vi "tripod gait (forNM)_0916.vi"(0 "data of 5th order formula\nts,tair,a1-a6":dbl[](array[numeric]), 1 "first or second":bool, 3 "buffer ratio":dbl, 4 "t_shift":dbl=0.000125, 5 "sample time":dbl=0.002, 9 "T_ratio":dbl, 10 "initial":bool) -> (7 "R1、R2 at 180":cluster{"1 at 180":bool, "2 at 180":bool}, 8 "reset step(indicator)":bool, 11 "start to calculate power":bool, 12 "output data":bool, 13 "Confirm(indicator)":bool, 14 "now gait info":T1, 15 "t1 out":dbl, 16 "finished":bool, 17 "t2 out":dbl, 18 "SET POINT V":dbl(graph), 19 "start to calculate the cost":bool, 20 "state":dbl, 21 "state 2":dbl, 23 "Set Point":dbl, 24 "Set Point 2":dbl, 25 "step count NM":dbl, 26 "period":dbl, 27 "new data of 5th NM":dbl[](array[numeric]))   [LabVIEW 2019]
panel:
  out "set point 2":dbl(graph)
  out "set point":dbl(graph)
  out "Numeric":dbl
  out "beta":dbl
  # "Nelder Mead"
  # "Input"
  # "Output"
  # "Others"
  # "loop period(ms)"
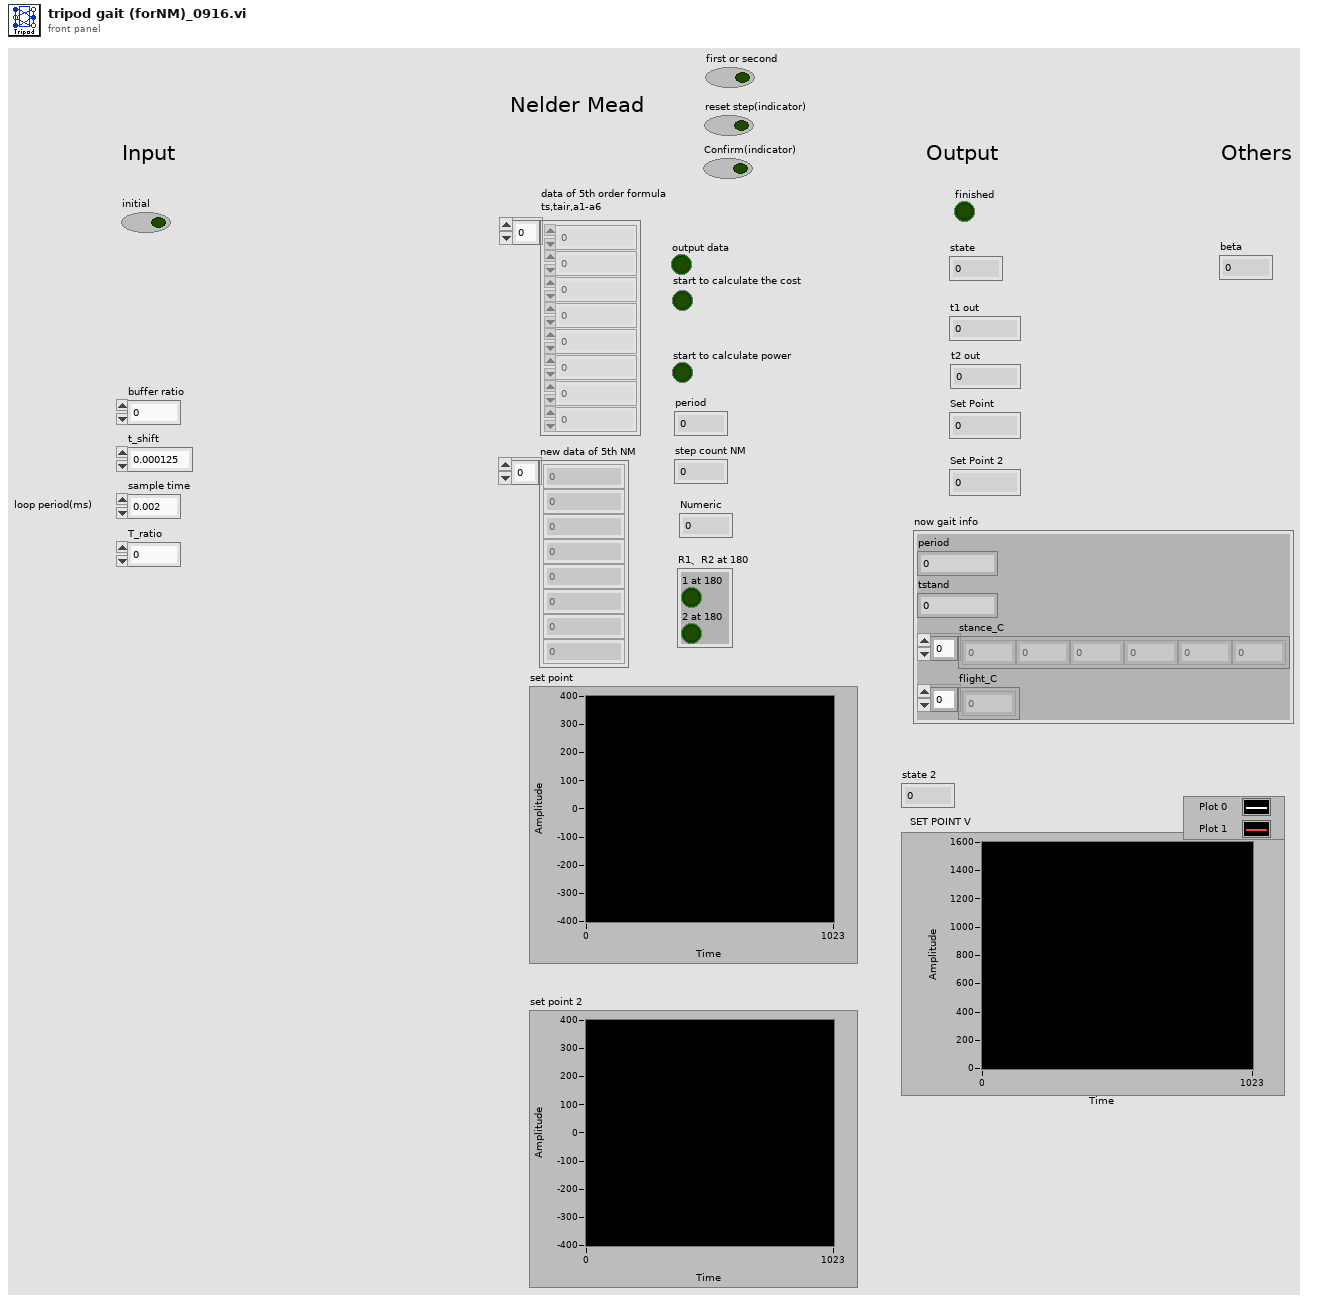
[diagram p1: front panel]
types:
  T1 = cluster{"period":dbl, "tstand":dbl, "stance_C":dbl[], "flight_C":dbl[]}
  T2 = cluster{"output cluster 2":cluster{"period":dbl, "tstand":dbl, "stance_C":dbl[], "flight_C":dbl[]}, "time180":dbl}
  T3 = cluster{"output cluster 2":cluster{"period":dbl, "tstand":dbl, "stance_C":dbl[], "flight_C":dbl[]}, "t2_out":dbl}
  T4 = cluster{"output cluster 2":cluster{"period":dbl, "tstand":dbl, "stance_C":dbl[], "flight_C":dbl[]}, "t1_out":dbl}
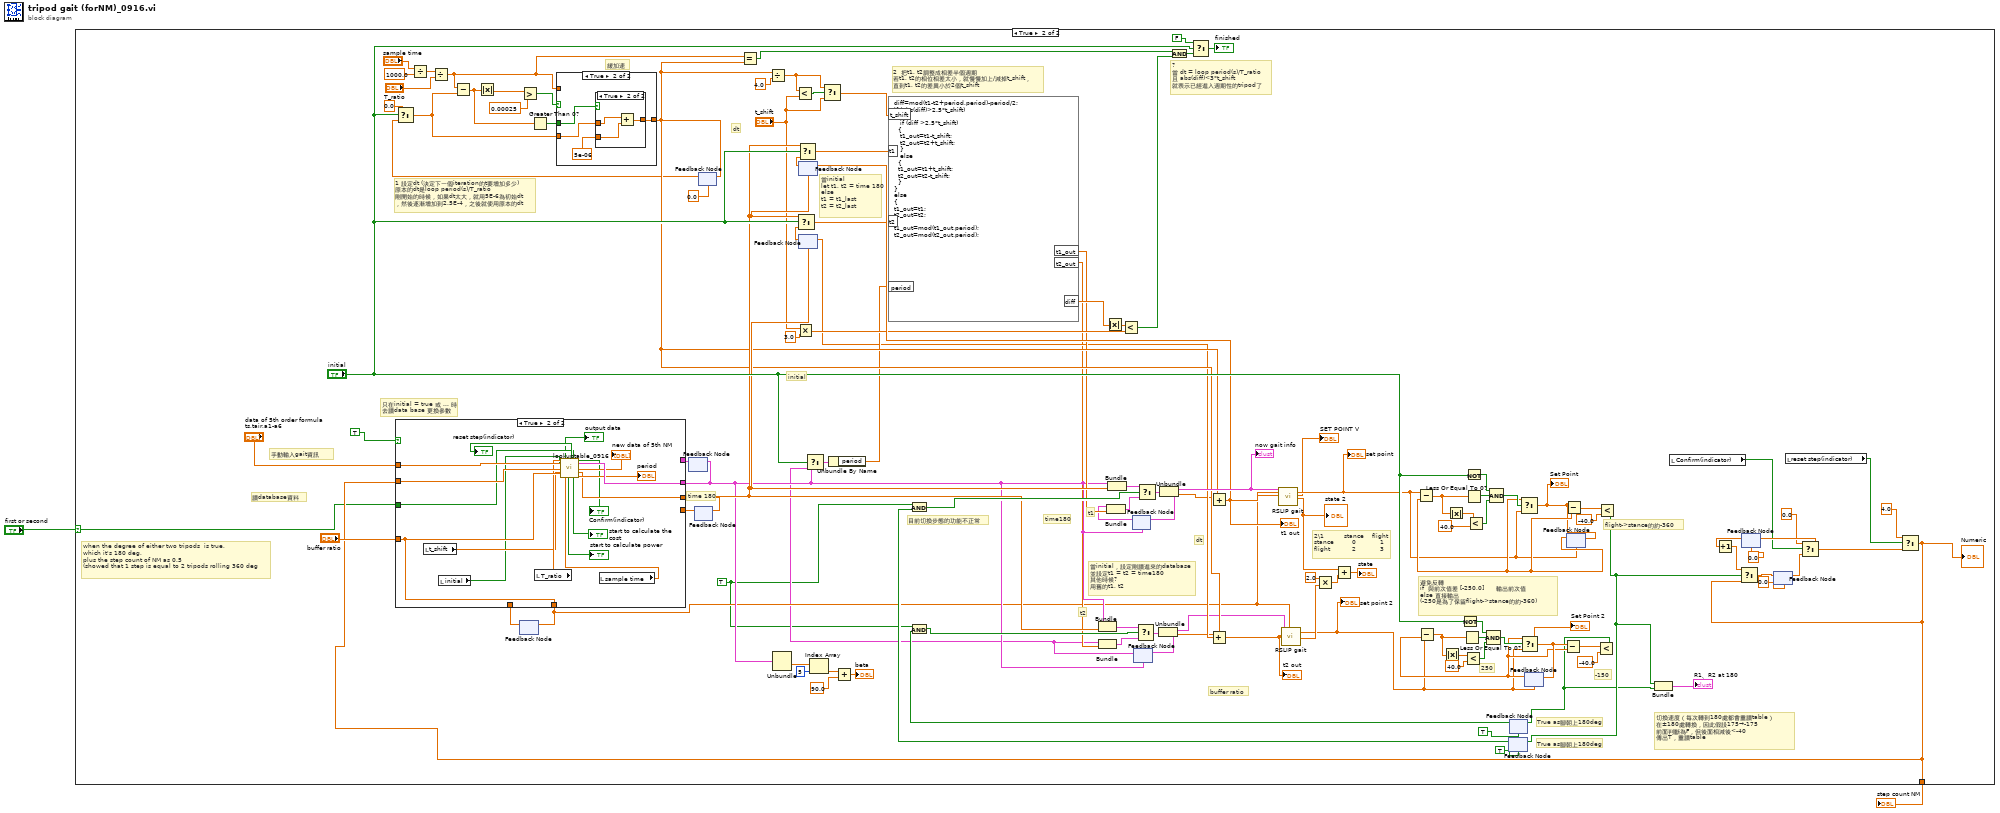
[diagram p0: block diagram]
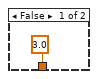
[diagram p2: hidden frame]
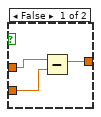
[diagram p4: hidden frame]
diagram:
  n1 = case shown="True" "first or second" {
    selector: "first or second" -> [_ w11]
    tunnel: [3.0 ("t") w13] -> w2
    frame False {
    }
    frame True {
      w31 = TRUE
      # "when the degree of either two tripods  is true, \nwhich it's 180 deg, \nplus the step count of NM as 0.5\n(showed that 1 step is equal to 2 tripods rolling 360 deg"
      # "目前切換步態的功能不正常"
      # "True as腳朝上180deg"
      # "True as腳朝上180deg"
      # "time180"
      # "t2"
      # "t1"
      # "dt"
      # "當initial，設定剛讀進來的database\n並設定t1 = t2 = time180\n其他時候?\n用舊的t1, t2"
      # "當initial\nlet t1, t2 = time 180\nelse\nt1 = t1_last\nt2 = t2_last"
      # "2  把t1, t2調整成相差半個週期\n若t1, t2的相位相差太小，就慢慢加上/減掉t_shift，\n直到t1, t2的差異小於2個t_shift"
      # "只在initial = true 或 ... 時\n去讀data base 更換參數"
      # "?\n當 dt = loop period(s)/T_ratio\n且 abs(diff)<3*t_shift\n就表示已經進入週期性的tripod了"
      # "1 設定dt (決定下一個iteration的t要增加多少)\n原本的dt是loop period(s)/T_ratio\n剛開始的時候，如果dt太大，就用5E-6為初始dt\n，然後逐漸增加到2.5E-4，之後就使用原本的dt"
      # "dt"
      # "initial"
      # "time 180"
      # "緩加速"
      # "切換速度（每次轉到180處都會重讀table）\n在±180處轉換，因此假設175→-175\n前面判斷為F，但後面相減後<-40\n傳出T，重讀table"
      # "手動輸入gait資訊"
      # "-150"
      # "250"
      # "buffer ratio"
      # "讀database資料"
      # "flight->stance的約-360"
      # "避免反轉\nif  與前次值差 [-250,0]      輸出前次值 \nelse 直接輸出\n(-250是為了保留flight->stance的約-360)"
      # "2\\1          stance    flight\nstance         0            1\nflight           2            3"
      n2 = Divide(x="sample time", y=1000.0) -> (x/y=w85:dbl)
      n3 = Divide(x=w85, y="T_ratio") -> (x/y=w86:dbl)
      n4 = feedback #1() -> (w105:dbl)  [unwired: 1 in]
      n5 = feedback #2() -> (w37:T1)  [unwired: 1 in]
      n6 = feedback #3() -> (w104:dbl)  [unwired: 1 in]
      n7 = feedback #4(0.0 ("sampling time")) -> (w73:dbl)
      n8 = Select(t=0.0, s="initial", f=w73) -> (s? t:f=w74:dbl)
      n9 = Subtract(x=w86, y=w74) -> (x-y=w88:dbl)
      n10 = Absolute Value(x=w88) -> (abs(x)=w71:dbl)
      n11 = Greater?(x=w71, y=0.00025) -> (0:w72:bool)
      n12 = Greater Than 0?(x=w88) -> (x > 0?=w89:bool)
      n13 = case shown="True" w72 {
        tunnel: w86 -> [w123 _]
        tunnel: [w123 w126] -> w81
        tunnel: w74 -> [_ w127]
        tunnel: w89 -> [_ w125]
        frame False {
        }
        frame True {
          n14 = case shown="True" w125 {
            tunnel: w127 -> [w130 w132]
            tunnel: [w129 w133] -> w126
            tunnel: 5e-06 ("x") -> [w128 w131]
            frame False {
              n15 = Subtract(x=w130, y=w128) -> (x-y=w129:dbl)
            }
            frame True {
              n16 = Add(x=w132, y=w131) -> (x+y=w133:dbl)
            }
          }
        }
      }
      n17 = feedback-in #4(w81) -> ()
      n18 = Equal?(x=w86, y=w81) -> (x = y?=w82:bool)
      n19 = Divide(x=w81, y=4.0) -> (x/y=w76:dbl)
      n20 = Less?(x=w76, y="t_shift") -> (x < y?=w75:bool)
      n21 = Multiply(x="t_shift", y=3.0) -> (x*y=w106:dbl)
      n22 = Select(t=w76, s=w75, f="t_shift") -> (s? t:f=w77:dbl)
      n23 = Not(x="initial") -> (.not. x?=w100:bool)
      n24 = Not(x="initial") -> (.not. x?=w96:bool)
      n25 = feedback #5(TRUE) -> (w116:bool)
      n26 = And(x=w31, y=w116) -> (x .and. y?=w110:bool)
      n27 = feedback #6(TRUE) -> (w115:bool)
      n28 = And(x=w31, y=w115) -> (x .and. y?=w111:bool)
      n29 = local read "Confirm(indicator)"() -> (w120:bool)
      n30 = feedback #7(0.0) -> (w118:dbl)
      n31 = Increment(x=w118) -> (x+1=w117:dbl)
      n32 = feedback #8(0.0 ("t")) -> (w119:dbl)
      n33 = local read "reset step(indicator)"() -> (w122:bool)
      n34 = Select(t=0.0, s=w120, f=w119) -> (s? t:f=w121:dbl)
      n35 = feedback-in #7(w121) -> ()
      n36 = Select(t=4.0, s=w122, f=w121) -> (s? t:f=w13:dbl)
      "Numeric" <- w13
      n37 = case shown="True" TRUE {
        tunnel: "buffer ratio" -> [_ w153]
        tunnel: [w134 w145] -> w107
        tunnel: [w136 w152] -> w68
        tunnel: w37 -> [w136 _]
        tunnel: [w135 w153] -> w64
        tunnel: w104 -> [w134 _]
        tunnel: w105 -> [w135 _]
        tunnel: "data of 5th order formula\nts,tair,a1-a6" -> [_ w151]
        tunnel: w13 -> [_ w146]
        tunnel: w11 -> [_ w142]
        frame False {
        }
        frame True {
          n38 = local read "t_shift"() -> (w140:dbl)
          n39 = local read "initial"() -> (w137:bool)
          n40 = local read "T_ratio"() -> (w141:dbl)
          n41 = local read "sample time"() -> (w139:dbl)
          n42 = call "lookuptable_0916.vi"("T_ratio"=w141, "data of 5th order formula\nts,tair,a1-a6 \n(input from the main program)"=w151, "step count NM"=w146, "t_shift"=w140, "Sample time"=w139, "initial"=w137, "buffer ratio"=w153, "first or second"=w142) -> ("output data"=→"output data":bool, "reset step(indicator)"=→"reset step(indicator)":bool, "start to calculate the power"=→"start to calculate power":bool, "start to calculate the cost"=→"start to calculate the cost":bool, "Confirm(indicator)"=→"Confirm(indicator)":bool, "output cluster 2"=w152:T1, "new data of 5th NM"=→"new data of 5th NM":dbl[], "time180"=w145:dbl, "period"=→"period":dbl)  [unwired: 3 in]
        }
      }
      n43 = feedback-in #1(w64) -> ()
      n44 = feedback-in #2(w68) -> ()
      n45 = feedback-in #3(w107) -> ()
      n46 = Unbundle(w68) -> ("stance_C"=w57:dbl[])  [unwired: 3 out]
      n47 = feedback #9(w107) -> (w93:dbl)
      n48 = Select(t=w107, s="initial", f=w93) -> (s? t:f=w92:dbl)
      n49 = feedback #10(w107) -> (w94:dbl)
      n50 = Select(t=w107, s="initial", f=w94) -> (s? t:f=w95:dbl)
      n51 = Index Array(array=w57, index=5) -> (element=w58:dbl)
      n52 = Add(x=w58, y=90.0) -> (x+y=→"beta":dbl)
      n53 = Bundle("output cluster 2"=w68, "time180"=w107) -> (w49:T2)  [unwired: 1 in]
      n54 = Bundle("output cluster 2"=w68, "time180"=w107) -> (w44:T2)  [unwired: 1 in]
      n55 = feedback #11(w68) -> (w46:T1)
      n56 = feedback #12(w68) -> (w53:T1)
      n57 = Select(t=w68, s="initial", f=w53) -> (s? t:f=w54:T1)
      n58 = Unbundle By Name(w54) -> ("period"=w69:dbl)
      n59 = formula code="diff=mod(t1-t2+period,period)-period/2;\nif (abs(diff)>2.5*t_shift)\n{\n   if (diff >2.5*t_shift)\n  {\n   t1_out=t1-t_shift;\n   t2_out=t2+t_shift;\n   }\n   else \n  {\n  t1_out=t1+t_shift;\n  t2_out=t2-t_shift;\n  }\n}\nelse\n{\nt1_out=t1;\nt2_out=t2;\n}\nt1_out=mod(t1_out,period);\nt2_out=mod(t2_out,period);"("period"=w69, "t1"=w92, "t2"=w95, "t_shift"=w77) -> ("t1_out"=w70:dbl, "t2_out"=w66:dbl, "diff"=w80:dbl)
      n60 = Bundle("output cluster 2"=w53, "t2_out"=w66) -> (w50:T3)  [unwired: 1 in]
      n61 = Absolute Value(x=w80) -> (abs(x)=w79:dbl)
      n62 = Bundle("output cluster 2"=w46, "t1_out"=w70) -> (w47:T4)  [unwired: 1 in]
      n63 = Less?(x=w79, y=w106) -> (x < y?=w83:bool)
      n64 = Select(t=w49, s=w111, f=w50) -> (s? t:f=w48:T3)
      n65 = Select(t=w44, s=w110, f=w47) -> (s? t:f=w45:T4)
      n66 = Unbundle(w48) -> ("output cluster 2"=w62:T1, "t2_out"=w52:dbl)
      n67 = feedback-in #12(w62) -> ()
      n68 = Unbundle(w45) -> ("output cluster 2"=w112:T1, "t1_out"=w51:dbl)
      "now gait info" <- w112
      n69 = feedback-in #11(w112) -> ()
      n70 = And(x=w82, y=w83) -> (x .and. y?=w90:bool)
      n71 = Select(t=FALSE, s="initial", f=w90) -> (s? t:f=→"finished":bool)
      n72 = Add(x=w52, y=w81) -> (x+y=w67:dbl)
      "t2 out" <- w67
      n73 = feedback-in #10(w67) -> ()
      n74 = Add(x=w51, y=w81) -> (x+y=w108:dbl)
      "t1 out" <- w108
      n75 = feedback-in #9(w108) -> ()
      n76 = call "RSLIP gait.vi"("gait Data"=w112, "Buffer Ratio"=w64, "Input Time"=w108) -> ("Set Point"=w10:dbl, "Set Point (V)"=→"SET POINT V":dbl, "state"=w61:dbl)  [unwired: 13 in, 1 out]
      "set point" <- w10
      "state 2" <- w61
      n77 = call "RSLIP gait.vi"("gait Data"=w62, "Buffer Ratio"=w64, "Input Time"=w67) -> ("Set Point"=w9:dbl, "state"=w63:dbl)  [unwired: 13 in, 2 out]
      "set point 2" <- w9
      n78 = Multiply(x=2.0, y=w63) -> (x*y=w56:dbl)
      n79 = Add(x=w61, y=w56) -> (x+y=→"state":dbl)
      n80 = feedback #13(w9) -> (w60:dbl)
      n81 = Subtract(x=w9, y=w60) -> (x-y=w41:dbl)
      n82 = Absolute Value(x=w41) -> (abs(x)=w42:dbl)
      n83 = Less Or Equal To 0?(x=w41) -> (x <= 0?=w101:bool)
      n84 = Less?(x=w42, y=40.0) -> (x < y?=w102:bool)
      n85 = Compound Arithmetic op=AND(w100, w101, w102) -> (w103:bool)
      n86 = Select(t=w60, s=w103, f=w9) -> (s? t:f=w114:dbl)
      "Set Point 2" <- w114
      n87 = feedback-in #13(w114) -> ()
      n88 = Subtract(x=w114, y=w60) -> (x-y=w43:dbl)
      n89 = feedback #14(w10) -> (w65:dbl)
      n90 = Subtract(x=w10, y=w65) -> (x-y=w39:dbl)
      n91 = Absolute Value(x=w39) -> (abs(x)=w40:dbl)
      n92 = Less Or Equal To 0?(x=w39) -> (x <= 0?=w97:bool)
      n93 = Less?(x=w40, y=40.0) -> (x < y?=w98:bool)
      n94 = Compound Arithmetic op=AND(w96, w97, w98) -> (w99:bool)
      n95 = Select(t=w65, s=w99, f=w10) -> (s? t:f=w4:dbl)
      "Set Point" <- w4
      n96 = Subtract(x=w4, y=w65) -> (x-y=w38:dbl)
      n97 = feedback-in #14(w4) -> ()
      n98 = Less?(x=w43, y=-40.0) -> (x < y?=w7:bool)
      n99 = feedback-in #6(w7) -> ()
      n100 = Less?(x=w38, y=-40.0) -> (x < y?=w8:bool)
      n101 = feedback-in #5(w8) -> ()
      n102 = Bundle(w8, w7) -> (→"R1、R2 at 180":cluster{bool, bool})  [unwired: 1 in]
      n103 = Select(t=w117, s=w8, f=w13) -> (s? t:f=w12:dbl)
      n104 = feedback-in #8(w12) -> ()
    }
  }
  "step count NM" <- w2
